vi "get_featurestudio_features.vi"(0 "Device In":T1, 11 "Error in":errorcluster) -> (4 "Device Out":T1, 6 "Comm":T2, 15 "Error Out":errorcluster)   [LabVIEW 2019]
uses:
  <userlib>/IoT Devices/_subVIs/HTTPComm.ctl
  <userlib>/Onshape/_SubVI/Cluster.ctl
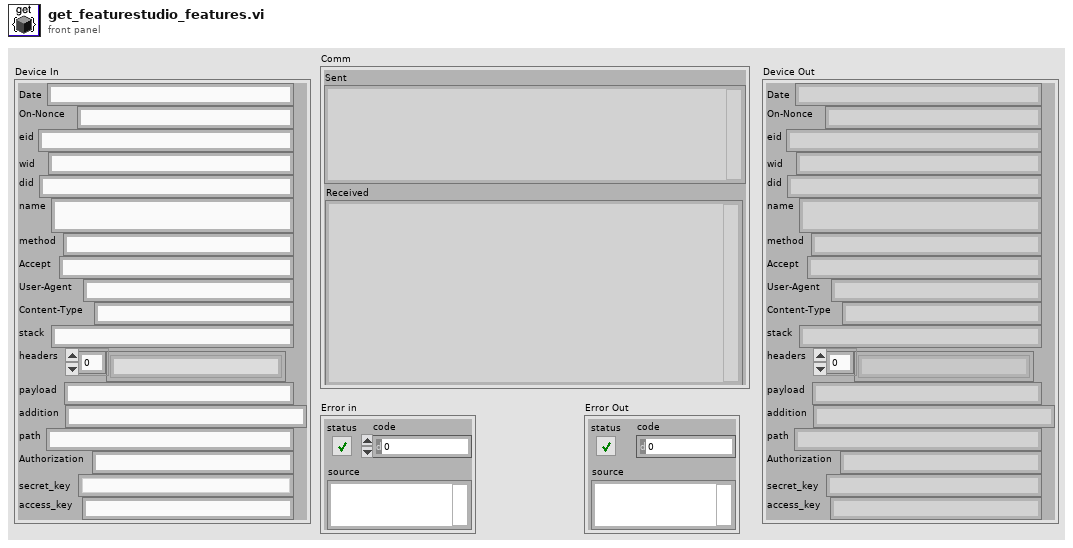
[diagram p1: front panel]
types:
  T1 = typedef "Cluster.ctl" = cluster{"Date":string, "On-Nonce":string, "eid":string, "wid":string, "did":string, "name":string, "method":string, "Accept":string, "User-Agent":string, "Content-Type":string, "stack":string, "headers":string[], "payload":string, "addition":string, "path":string, "Authorization":string, "secret_key":string, "access_key":string}
  T2 = typedef "HTTPComm.ctl" = cluster{"url":string, "sent headers":string, "sent body":string, "headers":string, "body":string, "Sent":string, "Received":string}
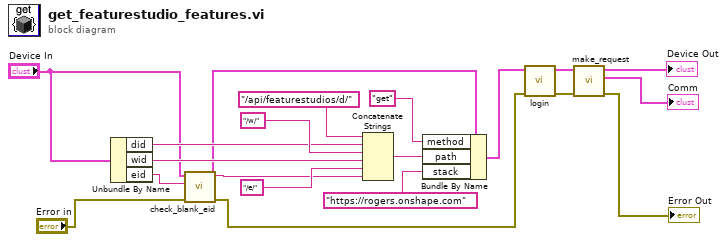
[diagram p0: block diagram]
diagram:
  n1 = Unbundle By Name("Device In") -> ("did"=w11:string, "wid"=w10:string, "eid"=w6:string)
  n2 = call <userlib>:"check_blank_eid.vi"("error in (no error)"="Error in", "eid in"=w6, "Device In"="Device In") -> ("error out"=w3:errorcluster, "Device Out"=w1:T1, "eid out"=w5:string)  [unwired: 6 in]
  n3 = Concatenate Strings("/api/featurestudios/d/" ("payload"), w11, "/w/" ("string"), w10, "/e/" ("string"), w5) -> (w16:string)
  n4 = Bundle By Name(cluster=w1, "method"="get" ("Method"), "path"=w16, "stack"="https://rogers.onshape.com" ("stacks")) -> (w13:T1)
  n5 = call <userlib>:"login.vi"("error in"=w3, "Device In"=w13) -> ("error out"=w12:errorcluster, "Device Out"=w14:T1)  [unwired: 8 in]
  n6 = call <userlib>:"make_request.vi"("Error in"=w12, "Device In"=w14) -> ("error out"=→"Error Out":errorcluster, "Comm"=→"Comm":T2, "Device Out"=→"Device Out":T1)  [unwired: 5 in, 2 out]
